vi "main.vi"() -> ()   [LabVIEW 2019]
uses:
  <vilib>/Utility/sysdir.llb/System Directory Type.ctl
  <vilib>/Platform/browser.llb/Open URL in Default Browser (string).vi
  <vilib>/Utility/cursorutil.llb/Set Cursor (Icon Pict).vi
  <vilib>/regexp/Match Regular Expression.xnode
  lib/libSimulationControl/libSimulationControl.lvlib
panel:
  out "Impressum":string
  out "Running?":bool
  in  "Help Button":bool
  in  "Break":bool
  in  "Plot":bool
  in  "Stop Button":bool
  in  "Pause Button":bool
  in  "Run":bool
  in  "Tab Control":T1(tab)
  out "Active element":string
  out "Iteration":i32
  out "Plant structure":string
  out "Simulation log":string
  in  "Auto Scroll":bool
  in  "Reset":bool
  in  "Uncouple":bool
  out "Working directory":path
  out "Runtime":dbl
  in  "Console":bool
  out "Runtime":string
  in  "Env. Clear":bool
  out "Env. Structure":string
  in  "Load Env":bool
  out "Environtment ready?":bool
  in  "Create Env":bool
  in  "Environtment Dir":path
  in  "Environment Tree":string(tree)
  out "Reactor Legend":picture
  in  "Show legend":bool
  out "Feedback?":bool
  out "Methane?":bool
  out "Storage?":bool
  out "#Hydrolysis":dbl
  out "Plant":picture
  in  "Reactor State":string(combo)="STRUCT_1_STAGE.vi"
  in  "Flow [L/h]":dbl=10.0 min=5.0 max=100.0 step=1.0
  in  "Hydrolysis specification":path
  in  "Methane specification":path
  in  "Auto cleanup?":bool
  in  "Endtime":dbl
  in  "Starttime":dbl
  in  "Edit Methane":bool
  in  "Edit Hydro":bool
  in  "Simulation file":path
  out "#Reactors":i32
  in  "Inflow fractions":T2(array[cluster]) {"Vertical Pointer Slide" scale=0.0..100.0 scale format="%.0f%"}
  in  "Hydrolysis PH":cluster{"Meter":dbl, "String":string}[][](array[cluster]) {"Meter" scale=0.0..14.0}
  in  "Load Feeding":bool
  in  "Save Feeding":bool
  out "Valid stamp?":bool
  out "Next timestep":dbl
  in  "Reactor":string(combo)
  in  "Delete":bool
  in  "Add timestamp":string[](array[string])
  in  "Add":bool
  in  "Feeding table":i32(listbox)
  out "timetable":string
  # "Biogas simulation Control"
  # "Before you start the simulation you need to set up a working environment.\nThe environment will be for the chosen reactor structure only."
  # "If you want the hydrolysis reactors to start with different initial values, you need to set up a working environtment first."
  # "Change the proportions at which the methane outflow will \nbe fed back into the hydrolysis reactors:"
  # "Add feeding hours and amount for a hydrolysis reactor."
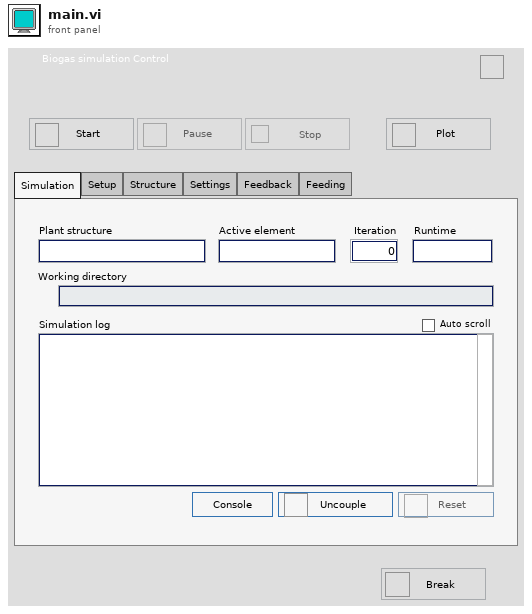
[diagram p1: front panel]
types:
  T1 = enum32{"Simulation", "Setup", "Structure", "Settings", "Feedback", "Feeding"}
  T2 = cluster{"Vertical Pointer Slide":i32, "String":string}[]
  T3 = typedef "System Directory Type.ctl" = i32
  T4 = enum8{"Enabled", "Disabled", "Disabled and Grayed Out"}
  T5 = typedef "LVPoint32TypeDef.ctl" = cluster{"Horizontal":i32, "Vertical":i32}
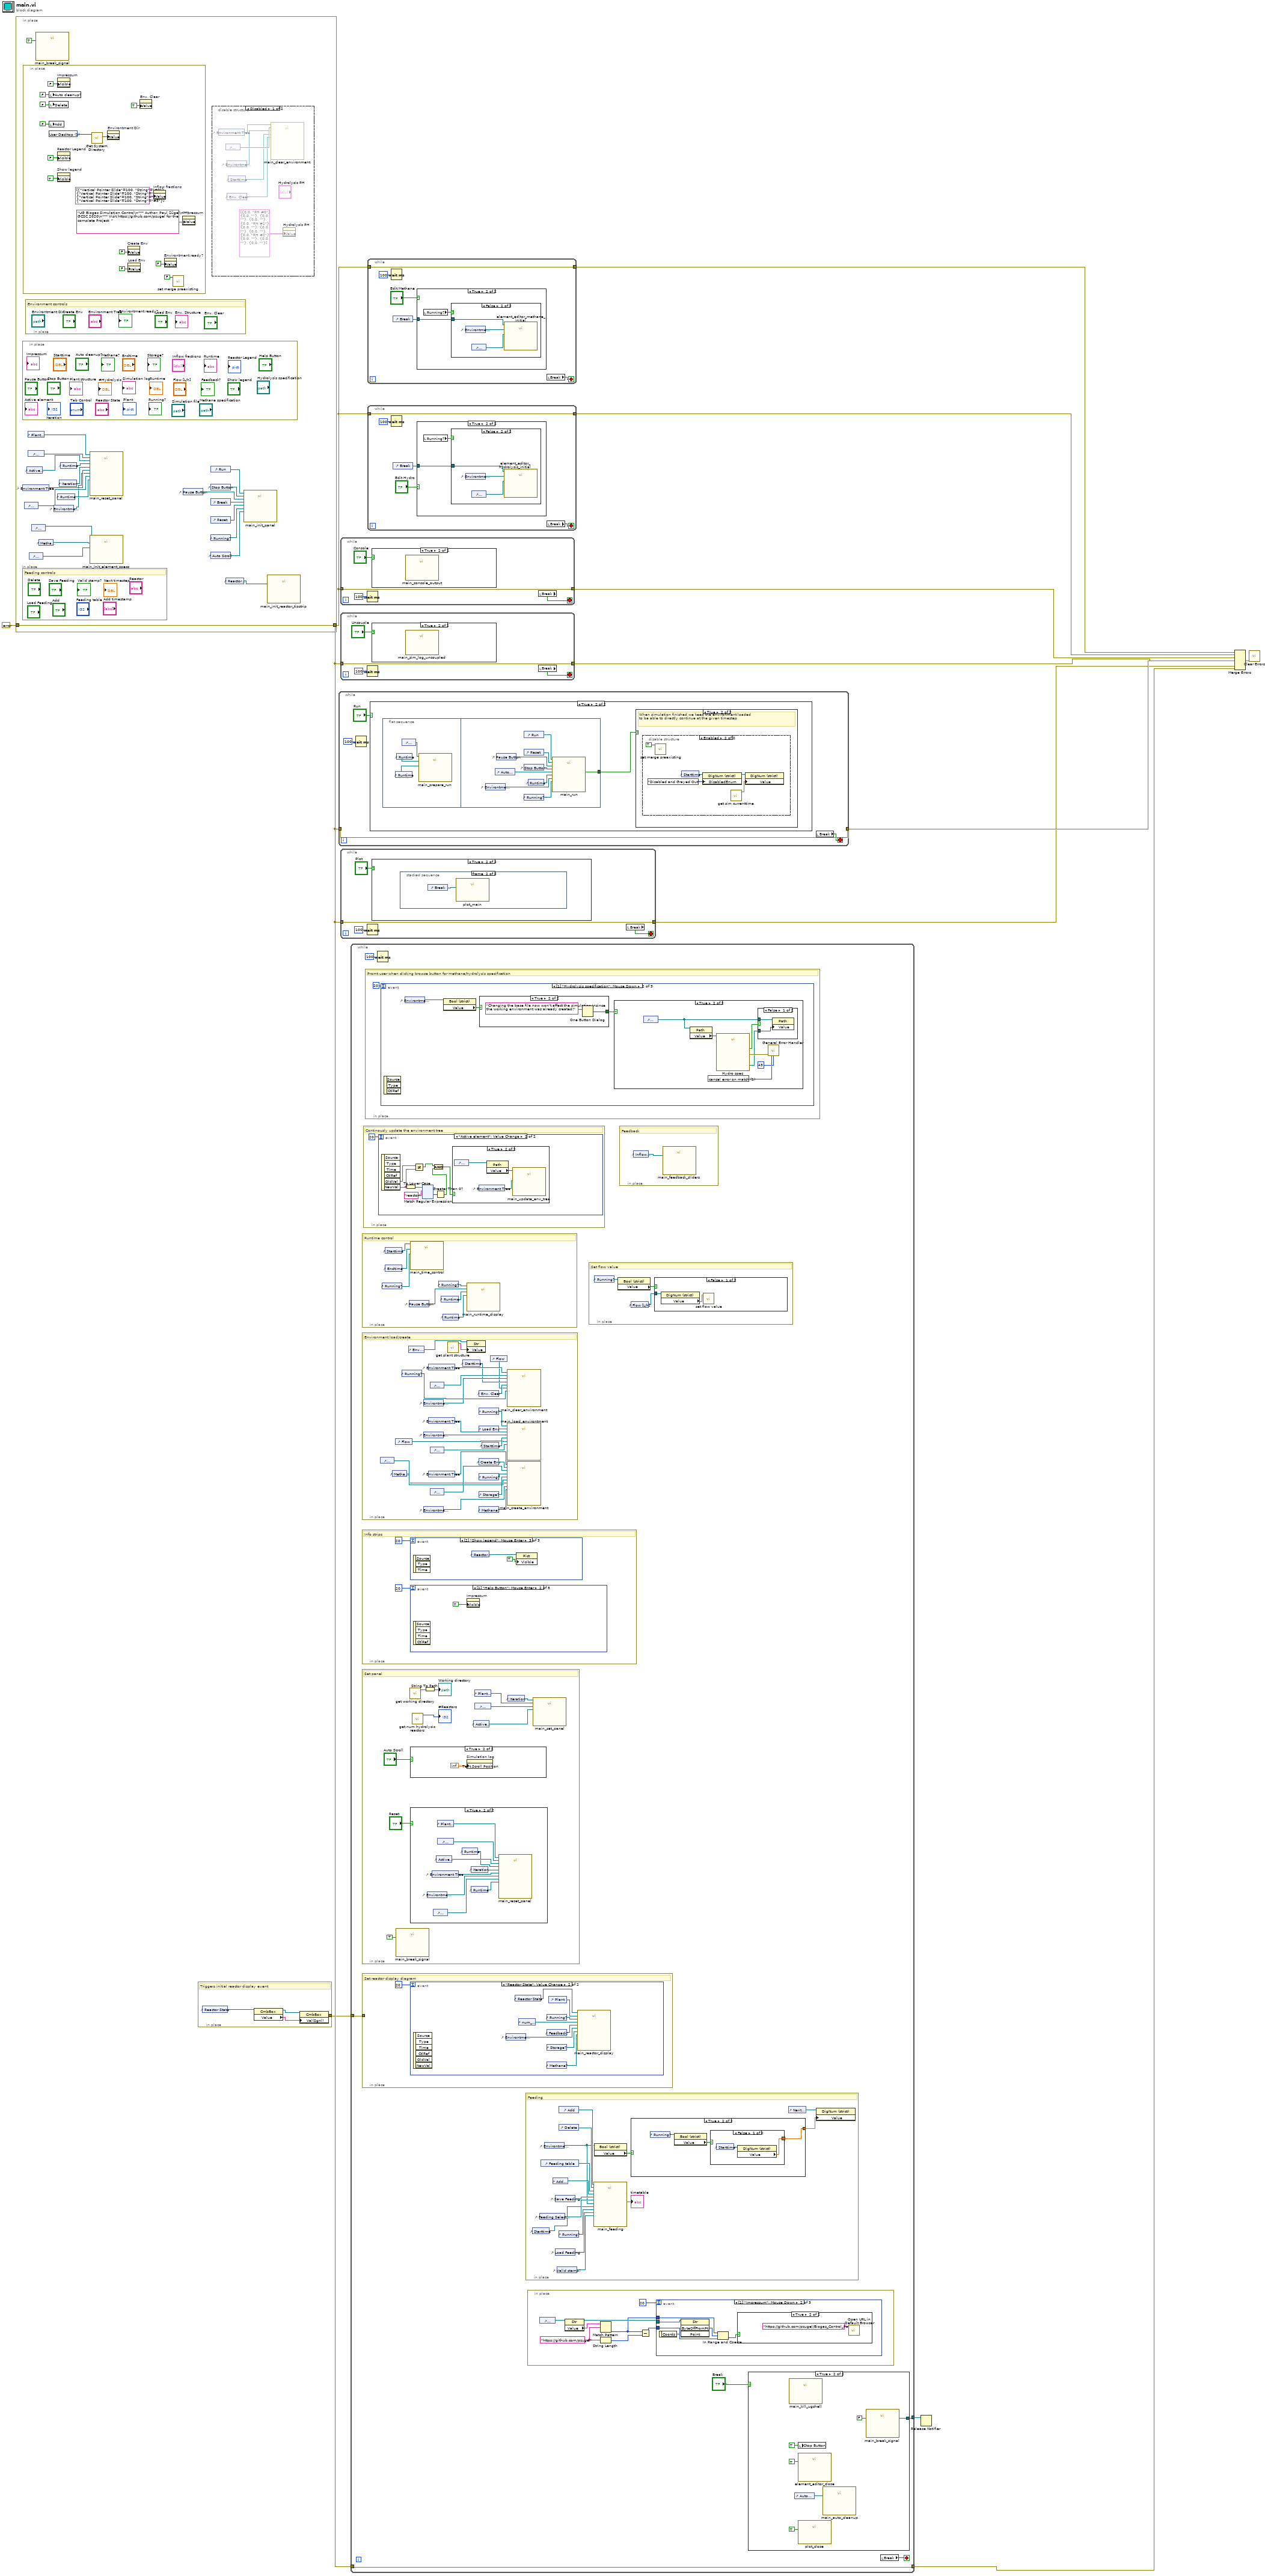
[diagram p0: block diagram]
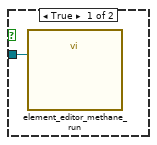
[diagram p3: hidden frame]
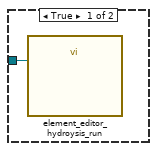
[diagram p5: hidden frame]
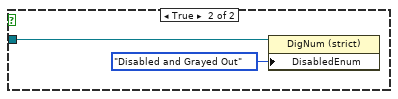
[diagram p8: hidden frame]
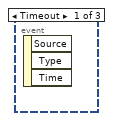
[diagram p9: hidden frame]
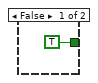
[diagram p10: hidden frame]
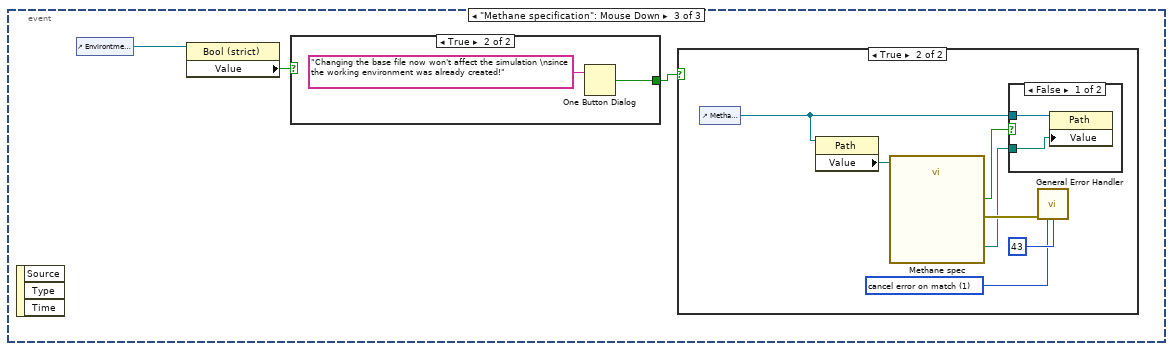
[diagram p13: hidden frame]
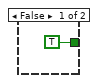
[diagram p16: hidden frame]
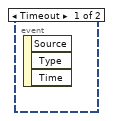
[diagram p17: hidden frame]
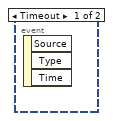
[diagram p19: hidden frame]
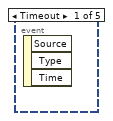
[diagram p20: hidden frame]
diagram:
  n1 = in-place {
    in-place-border: [w34] -> w5
    in-place-border: errorcluster {"status"=FALSE, "code"=0, "source"=""} ("error constant") -> [w34]
    n2 = in-place {
    }
    n3 = control-ref of="Environment Tree"() -> (w17:refnum<vi>)
    n4 = in-place {
      # "Feeding controls"
    }
    n5 = in-place {
      w46 = T3 1 items=["User Home"=0, "User Desktop"=1, "User Documents"=2, "User Application Data"=3, "User Preferences"=4, "User Temporary"=5, "Public Documents"=6, "Public Application Data"=7, "Public Preferences"=8, "Public Cache"=13, "System Core Libraries"=9, "System Installed Libraries"=10, "Application Files"=11, "Boot Volume Root"=12] ("system directory type")
      n6 = local write "Auto cleanup?"(FALSE ("Auto Cleanup?")) -> ()
      n7 = local write "Delete"(FALSE ("Delete")) -> ()
      n8 = local write "Add"(FALSE ("Add")) -> ()
      n9 = property on="Impressum" class="Str"("Visible"=FALSE) -> ()  [unwired: 2 in, 2 out]
      n10 = property on="Reactor Legend" class="Pict"("Visible"=FALSE) -> ()  [unwired: 2 in, 2 out]
      n11 = property on="Show legend" class="Bool"("Visible"=TRUE) -> ()  [unwired: 2 in, 2 out]
      n12 = call <vilib>:"Get System Directory.vi"("system directory type"=w46) -> ("system directory"=w47:path)  [unwired: 10 in]
      n13 = property on="Environtment Dir" class="Path"("Value"=w47) -> ()  [unwired: 2 in, 2 out]
      n14 = property on="Create Env" class="Bool (strict)"("Value"=FALSE ("Create Env")) -> ()  [unwired: 2 in, 2 out]
      n15 = property on="Load Env" class="Bool (strict)"("Value"=FALSE ("Load Env")) -> ()  [unwired: 2 in, 2 out]
      n16 = property on="Env. Clear" class="Bool (strict)"("Value"=TRUE ("Env. Clear")) -> ()  [unwired: 2 in, 2 out]
      n17 = property on="Inflow fractions" class="Arr (strict)"("Value"=T2 [{"Vertical Pointer Slide"=100, "String"="#0"}, {"Vertical Pointer Slide"=100, "String"="#1"}, {"Vertical Pointer Slide"=100, "String"="#2"}, {"Vertical Pointer Slide"=100, "String"="#3"}] ("Inflow fractions")) -> ()  [unwired: 2 in, 2 out]
      n18 = property on="Environtment ready?" class="Bool (strict)"("Value"=FALSE ("Environtment ready?")) -> ()  [unwired: 2 in, 2 out]
      n19 = call "set merge preexisting.vi"("merge"=FALSE) -> ()  [unwired: 10 in, 1 out]
      n20 = property on="Impressum" class="Str"("Value"="UG Biogas Simulation Control\n*** Author: Paul Zügel\n*** GCSC 2020\n*** Visit https://github.com/pzugel for the complete Project  " ("String")) -> ()  [unwired: 2 in, 2 out]
    }
    n21 = control-ref of="Environtment Dir"() -> (w18:refnum<vi>)
    n22 = in-place {
      # "Environment controls"
    }
    n23 = control-ref of="Active element"() -> (w32:refnum<vi>)
    n24 = control-ref of="Plant structure"() -> (w30:refnum<vi>)
    n25 = control-ref of="Simulation log"() -> (w31:refnum<vi>)
    n26 = control-ref of="Simulation file"() -> (w20:refnum<vi>)
    n27 = control-ref of="Hydrolysis specification"() -> (w14:refnum<vi>)
    n28 = call "main_break_signal.vi"("Keep Running?"=TRUE ("Checkbox")) -> ()  [unwired: 10 in, 1 out]
    n29 = control-ref of="Methane specification"() -> (w13:refnum<vi>)
    n30 = control-ref of="Environtment ready?"() -> (w16:refnum<vi>)
    n31 = control-ref of="Runtime"() -> (w21:refnum<vi>)
    n32 = control-ref of="Iteration"() -> (w33:refnum<vi>)
    n33 = control-ref of="Runtime"() -> (w19:refnum<vi>)
    n34 = call "main_reset_panel.vi"("Env ready?"=w16, "Envi. Tree"=w17, "Env. Directory"=w18, "Iteration"=w33, "Runtime"=w21, "Runtime (string)"=w19, "Active Element"=w32, "Simulation Log"=w31, "Plant Structure"=w30) -> ()  [unwired: 3 in]
    n35 = call "main_init_element_specs.vi"("Simulation"=w20, "Methane"=w13, "Hydrolyse"=w14) -> ()  [unwired: 9 in]
    n36 = control-ref of="Pause Button"() -> (w23:refnum<vi>)
    n37 = control-ref of="Run"() -> (w29:refnum<vi>)
    n38 = control-ref of="Stop Button"() -> (w24:refnum<vi>)
    n39 = control-ref of="Break"() -> (w27:refnum<vi>)
    n40 = control-ref of="Reset"() -> (w28:refnum<vi>)
    n41 = control-ref of="Running?"() -> (w22:refnum<vi>)
    n42 = control-ref of="Auto Scroll"() -> (w26:refnum<vi>)
    n43 = disable-structure shown="Disabled" {
      frame Disabled {
        n44 = control-ref of="Environment Tree"() -> (w40:refnum<vi>)
        n45 = control-ref of="Environtment Dir"() -> (w39:refnum<vi>)
        n46 = control-ref of="Environtment ready?"() -> (w38:refnum<vi>)
        n47 = control-ref of="Env. Clear"() -> (w36:refnum<vi>)
        n48 = control-ref of="Starttime"() -> (w37:refnum<vi>)
        n49 = call "main_clear_environment.vi"("Env. Clear"=w36, "Starttime"=w37, "Env. ready?"=w38, "Env. Dir"=w39, "Env. Tree"=w40) -> ()  [unwired: 7 in]
        n50 = property on="Hydrolysis PH" class="Arr (strict)"("Value"=cluster{"Meter":dbl, "String":string}[][] [[{"Meter"=0.0, "String"="PH #0"}, {"Meter"=0.0, "String"=""}, {"Meter"=0.0, "String"=""}, {"Meter"=0.0, "String"=""}], [{"Meter"=0.0, "String"="PH #1"}, {"Meter"=0.0, "String"=""}, {"Meter"=0.0, "String"=""}, {"Meter"=0.0, "String"=""}], [{"Meter"=0.0, "String"="PH #2"}, {"Meter"=0.0, "String"=""}, {"Meter"=0.0, "String"=""}, {"Meter"=0.0, "String"=""}]] ("Hydrolysis PH")) -> ()  [unwired: 2 in, 2 out]
      }
      frame Enabled {
      }
    }
    n51 = control-ref of="Reactor Legend"() -> (w15:refnum<vi>)
    n52 = call "main_init_panel.vi"("Running?"=w22, "Reset"=w28, "Auto Scroll"=w26, "Break Button"=w27, "Pause Button"=w23, "Stop Button"=w24, "Run"=w29) -> ()  [unwired: 5 in]
    n53 = call "main_init_reactor_tipstrip.vi"("Reactor legend"=w15) -> ()  [unwired: 11 in]
  }
  n54 = in-place {
    in-place-border: [w56] -> w1
    # "Triggers initial reactor display event"
    n55 = control-ref of="Reactor State"() -> (w59:refnum<vi>)
    n56 = property class="CmbBox"(reference=w59) -> (reference out=w57:refnum<vi>, "Value"=w58:string)  [unwired: 1 in, 1 out]
    n57 = property class="CmbBox"(reference=w57, "Val(Sgnl)"=w58) -> (error out=w56:errorcluster)  [unwired: 1 in, 1 out]
  }
  n58 = while {
    tunnel: w5 -> [w63]
    tunnel: [w63] -> w11
    stop <- w61 stop-if-true
    n59 = Wait (ms)(milliseconds to wait=u32 100) -> ()  [unwired: 1 out]
    n60 = case shown="True" "Run" {
      frame False {
        n61 = property on="Run" class="Bool"("DisabledEnum"=T4."Enabled" ("Disabled")) -> ()  [unwired: 2 in, 2 out]
        n62 = property on="Stop Button" class="Bool (strict)"("DisabledEnum"=T4."Disabled and Grayed Out" ("Disabled")) -> ()  [unwired: 2 in, 2 out]
        n63 = property on="Pause Button" class="Bool (strict)"("DisabledEnum"=T4."Disabled and Grayed Out" ("Disabled")) -> ()  [unwired: 2 in, 2 out]
      }
      frame True {
        n64 = flat-sequence {
          tunnel: [w82] -> w67
          frame #0 {
            n65 = control-ref of="Runtime"() -> (w81:refnum<vi>)
            n66 = control-ref of="Runtime"() -> (w80:refnum<vi>)
            n67 = control-ref of="Environtment Dir"() -> (w79:refnum<vi>)
            n68 = call "main_prepare_run.vi"("Runtime"=w81, "Runtime String"=w80, "Env. Dir"=w79) -> ()  [unwired: 9 in]
          }
          frame #1 {
            n69 = control-ref of="Environtment ready?"() -> (w90:refnum<vi>)
            n70 = control-ref of="Auto cleanup?"() -> (w89:refnum<vi>)
            n71 = control-ref of="Pause Button"() -> (w86:refnum<vi>)
            n72 = control-ref of="Run"() -> (w84:refnum<vi>)
            n73 = control-ref of="Reset"() -> (w88:refnum<vi>)
            n74 = control-ref of="Stop Button"() -> (w85:refnum<vi>)
            n75 = control-ref of="Running?"() -> (w87:refnum<vi>)
            n76 = control-ref of="Runtime"() -> (w83:refnum<vi>)
            n77 = call "main_run.vi"("Runtime String"=w83, "Env ready?"=w90, "Cleanup?"=w89, "Running?"=w87, "Stop Button"=w85, "Pause Button"=w86, "Reset"=w88, "Run"=w84) -> ("OK?"=w82:bool)  [unwired: 3 in]
          }
        }
        n78 = case shown="True" w67 {
          frame False {
          }
          frame True {
            # "When simulation finished we keep the environment loaded\nto be able to directly continue at the given timestep"
            n79 = disable-structure shown="Enabled" {
              frame Disabled {
                n80 = control-ref of="Env. Clear"() -> (w72:refnum<vi>)
                n81 = property class="Bool (strict)"(reference=w72, "Value"=TRUE) -> (reference out=w73:refnum<vi>)  [unwired: 1 in, 1 out]
                n82 = control-ref of="Environtment ready?"() -> (w71:refnum<vi>)
                n83 = control-ref of="Environment Tree"() -> (w69:refnum<vi>)
                n84 = control-ref of="Environtment Dir"() -> (w70:refnum<vi>)
                n85 = call "main_clear_environment.vi"("Env. Clear"=w73, "Env. ready?"=w71, "Env. Dir"=w70, "Env. Tree"=w69) -> ()  [unwired: 8 in]
              }
              frame Enabled {
                n86 = call "set merge preexisting.vi"("merge"=TRUE) -> ()  [unwired: 10 in, 1 out]
                n87 = control-ref of="Starttime"() -> (w77:refnum<vi>)
                n88 = property class="DigNum (strict)"(reference=w77, "DisabledEnum"=T4."Disabled and Grayed Out" ("Disabled")) -> (reference out=w74:refnum<vi>)  [unwired: 1 in, 1 out]
                n89 = call "get sim currenttime.vi"() -> ("current_time"=w75:dbl)  [unwired: 10 in, 1 out]
                n90 = property class="DigNum (strict)"(reference=w74, "Value"=w75) -> ()  [unwired: 1 in, 2 out]
              }
            }
          }
        }
      }
    }
    n91 = local read "Break"() -> (w61:bool)
  }
  n92 = while {
    tunnel: w5 -> [w93]
    tunnel: [w93] -> w6
    stop <- w91 stop-if-true
    n93 = Wait (ms)(milliseconds to wait=u32 100) -> ()  [unwired: 1 out]
    n94 = case shown="True" "Console" {
      frame False {
      }
      frame True {
        n95 = call "main_console_output.vi"() -> ()  [unwired: 12 in]
      }
    }
    n96 = local read "Break"() -> (w91:bool)
  }
  n97 = while {
    tunnel: w5 -> [w97]
    tunnel: [w97] -> w7
    stop <- w95 stop-if-true
    n98 = Wait (ms)(milliseconds to wait=u32 100) -> ()  [unwired: 1 out]
    n99 = case shown="True" "Uncouple" {
      frame False {
      }
      frame True {
        n100 = call "main_sim_log_uncoupled.vi"() -> ()  [unwired: 12 in]
      }
    }
    n101 = local read "Break"() -> (w95:bool)
  }
  n102 = while {
    tunnel: w5 -> [w101]
    tunnel: [w101] -> w10
    stop <- w99 stop-if-true
    n103 = Wait (ms)(milliseconds to wait=u32 100) -> ()  [unwired: 1 out]
    n104 = case shown="True" "Plot" {
      frame False {
      }
      frame True {
        n105 = stacked-sequence {
          frame #0 {
            n106 = call "plot_close.vi"("Close?"=TRUE) -> ()  [unwired: 11 in]
          }
          frame #1 {
            n107 = control-ref of="Break"() -> (w104:refnum<vi>)
            n108 = call "plot_main.vi"("Break"=w104) -> ()  [unwired: 11 in]
          }
        }
      }
    }
    n109 = local read "Break"() -> (w99:bool)
  }
  n110 = while {
    tunnel: w5 -> [w110]
    tunnel: [w110] -> w9
    tunnel: [w108] -> w8
    tunnel: w1 -> [w105]
    stop <- w106 stop-if-true
    n111 = in-place {
      # "Runtime control"
      n112 = control-ref of="Running?"() -> (w280:refnum<vi>)
      n113 = control-ref of="Starttime"() -> (w282:refnum<vi>)
      n114 = control-ref of="Endtime"() -> (w281:refnum<vi>)
      n115 = control-ref of="Pause Button"() -> (w277:refnum<vi>)
      n116 = call "main_time_control.vi"("Running?"=w280, "Endtime"=w281, "Starttime"=w282) -> ()  [unwired: 9 in]
      n117 = control-ref of="Running?"() -> (w276:refnum<vi>)
      n118 = control-ref of="Runtime"() -> (w278:refnum<vi>)
      n119 = control-ref of="Runtime"() -> (w279:refnum<vi>)
      n120 = call "main_runtime_display.vi"("Runtime (string)"=w279, "Runtime"=w278, "Pause Button"=w277, "Running?"=w276) -> ()  [unwired: 8 in]
    }
    n121 = in-place {
      # "Environment load/create"
      n122 = control-ref of="Hydrolysis specification"() -> (w327:refnum<vi>)
      n123 = control-ref of="Methane specification"() -> (w326:refnum<vi>)
      n124 = control-ref of="Flow"() -> (w324:refnum<vi>)
      n125 = control-ref of="Running?"() -> (w325:refnum<vi>)
      n126 = control-ref of="Env. Structure"() -> (w337:refnum<vi>)
      n127 = control-ref of="Environtment ready?"() -> (w333:refnum<vi>)
      n128 = control-ref of="Environtment ready?"() -> (w336:refnum<vi>)
      n129 = control-ref of="Environtment ready?"() -> (w341:refnum<vi>)
      n130 = control-ref of="Environment Tree"() -> (w331:refnum<vi>)
      n131 = control-ref of="Environment Tree"() -> (w338:refnum<vi>)
      n132 = control-ref of="Environment Tree"() -> (w347:refnum<vi>)
      n133 = control-ref of="Environtment Dir"() -> (w332:refnum<vi>)
      n134 = control-ref of="Environtment Dir"() -> (w335:refnum<vi>)
      n135 = control-ref of="Environtment Dir"() -> (w345:refnum<vi>)
      n136 = call "get plant structure.vi"() -> ("function return"=w329:string)  [unwired: 10 in, 1 out]
      n137 = control-ref of="Starttime"() -> (w328:refnum<vi>)
      n138 = property class="Str"(reference=w337, "Value"=w329) -> ()  [unwired: 1 in, 2 out]
      n139 = control-ref of="Env. Clear"() -> (w334:refnum<vi>)
      n140 = control-ref of="Running?"() -> (w340:refnum<vi>)
      n141 = control-ref of="Load Env"() -> (w339:refnum<vi>)
      n142 = control-ref of="Create Env"() -> (w346:refnum<vi>)
      n143 = control-ref of="Running?"() -> (w344:refnum<vi>)
      n144 = control-ref of="Storage?"() -> (w343:refnum<vi>)
      n145 = control-ref of="Methane?"() -> (w342:refnum<vi>)
      n146 = control-ref of="Starttime"() -> (w330:refnum<vi>)
      n147 = control-ref of="Flow"() -> (w323:refnum<vi>)
      n148 = call "main_clear_environment.vi"("Flow"=w323, "Env. Clear"=w334, "Running?"=w325, "Starttime"=w328, "Env. ready?"=w333, "Env. Dir"=w332, "Env. Tree"=w331) -> ()  [unwired: 5 in]
      n149 = call "main_load_environtment.vi"("Flow"=w324, "Starttime"=w330, "Env. Dir"=w335, "Env. Ready?"=w336, "Environtment Tree"=w338, "Load Env"=w339, "Running?"=w340) -> ()  [unwired: 5 in]
      n150 = call "main_create_environment.vi"("Meth. Path"=w326, "Hydr. Path"=w327, "Ready?"=w341, "Storage?"=w343, "Methane?"=w342, "Running?"=w344, "Directory"=w345, "Create"=w346, "Environtment Tree"=w347) -> ()  [unwired: 3 in]
    }
    n151 = in-place {
      # "Info strips"
      n152 = event shown="[2] \"Show legend\": Mouse Enter" {
        selector: _ -> [_ _ _]
        dyn-events: _ -> [_ _ _]
        timeout: 20 -> [_ _ _]
        event Timeout {
          n153 = event-data() -> ()  [unwired: 1 in, 3 out]
        }
        event "Show legend": Mouse Leave {
          n154 = event-data() -> ()  [unwired: 1 in, 3 out]
          n155 = control-ref of="Reactor Legend"() -> (w300:refnum<vi>)
          n156 = property class="Pict"(reference=w300, "Visible"=FALSE) -> ()  [unwired: 1 in, 2 out]
        }
        event "Show legend": Mouse Enter {
          n157 = event-data() -> ()  [unwired: 1 in, 3 out]
          n158 = control-ref of="Reactor Legend"() -> (w302:refnum<vi>)
          n159 = property class="Pict"(reference=w302, "Visible"=TRUE) -> ()  [unwired: 1 in, 2 out]
        }
      }
      n160 = event shown="[1] \"Help Button\": Mouse Enter" {
        selector: _ -> [_ _ _ _ _]
        dyn-events: _ -> [_ _ _ _ _]
        timeout: 20 -> [_ _ _ _ _]
        event Timeout {
          n161 = event-data() -> ()  [unwired: 1 in, 3 out]
        }
        event "Help Button": Mouse Enter {
          n162 = event-data() -> ()  [unwired: 1 in, 4 out]
          n163 = property on="Impressum" class="Str"("Visible"=TRUE) -> ()  [unwired: 2 in, 2 out]
        }
        event "Help Button": Mouse Leave {
          n164 = event-data() -> ()  [unwired: 1 in, 4 out]
          n165 = event shown="[0] Timeout" {
            selector: _ -> [_ _]
            dyn-events: _ -> [_ _]
            timeout: 20 -> [_ _]
            event Timeout {
              n166 = event-data() -> ()  [unwired: 1 in, 3 out]
              n167 = property on="Impressum" class="Str"("Visible"=FALSE) -> ()  [unwired: 2 in, 2 out]
            }
            event "Impressum": Mouse Enter {
              n168 = event-data() -> ()  [unwired: 1 in, 3 out]
              n169 = property on="Impressum" class="Str"("Visible"=TRUE) -> ()  [unwired: 2 in, 2 out]
            }
          }
        }
        event "Impressum": Mouse Enter {
          n170 = event-data() -> ()  [unwired: 1 in, 4 out]
        }
        event "Impressum": Mouse Leave {
          n171 = event-data() -> ()  [unwired: 1 in, 4 out]
          n172 = property on="Impressum" class="Str"("Visible"=FALSE) -> ()  [unwired: 2 in, 2 out]
        }
      }
    }
    n173 = in-place {
      # "Set panel"
      n174 = call "main_break_signal.vi"("Keep Running?"=TRUE) -> ()  [unwired: 10 in, 1 out]
      n175 = call "get working directory.vi"() -> ("function return"=w312:string)  [unwired: 10 in, 1 out]
      n176 = case shown="True" "Auto Scroll" {
        frame False {
        }
        frame True {
          n177 = property on="Simulation log" class="Str"("Text.Scroll Position"=inf) -> ()  [unwired: 2 in, 2 out]
        }
      }
      n178 = case shown="True" "Reset" {
        frame False {
        }
        frame True {
          n179 = control-ref of="Environtment ready?"() -> (w314:refnum<vi>)
          n180 = control-ref of="Environment Tree"() -> (w315:refnum<vi>)
          n181 = control-ref of="Environtment Dir"() -> (w316:refnum<vi>)
          n182 = control-ref of="Active element"() -> (w320:refnum<vi>)
          n183 = control-ref of="Plant structure"() -> (w321:refnum<vi>)
          n184 = control-ref of="Simulation log"() -> (w318:refnum<vi>)
          n185 = control-ref of="Runtime"() -> (w313:refnum<vi>)
          n186 = control-ref of="Iteration"() -> (w319:refnum<vi>)
          n187 = control-ref of="Runtime"() -> (w317:refnum<vi>)
          n188 = call "main_reset_panel.vi"("Env ready?"=w314, "Envi. Tree"=w315, "Env. Directory"=w316, "Iteration"=w319, "Runtime"=w317, "Runtime (string)"=w313, "Active Element"=w320, "Simulation Log"=w318, "Plant Structure"=w321) -> ()  [unwired: 3 in]
        }
      }
      n189 = call "get num hydrolysis reactors.vi"() -> ("function return"=→"#Reactors":i32)  [unwired: 10 in, 1 out]
      n190 = String To Path(string=w312) -> (path=→"Working directory":path)
      n191 = control-ref of="Active element"() -> (w306:refnum<vi>)
      n192 = control-ref of="Plant structure"() -> (w304:refnum<vi>)
      n193 = control-ref of="Simulation log"() -> (w305:refnum<vi>)
      n194 = control-ref of="Iteration"() -> (w303:refnum<vi>)
      n195 = call "main_set_panel.vi"("Active Element"=w306, "Simulation Log"=w305, "Plant Structure"=w304, "Iteration"=w303) -> ()  [unwired: 8 in]
    }
    n196 = in-place {
      in-place-border: w105 -> [_]
      # "Set reactor display diagram"
      n197 = event shown="[1] \"Reactor State\": Value Change" {
        selector: _ -> [_ _]
        dyn-events: _ -> [_ _]
        timeout: 20 -> [_ _]
        event Timeout {
          n198 = event-data() -> ()  [unwired: 1 in, 3 out]
        }
        event "Reactor State": Value Change {
          n199 = event-data() -> ()  [unwired: 1 in, 6 out]
          n200 = control-ref of="Environtment ready?"() -> (w291:refnum<vi>)
          n201 = control-ref of="Reactor State"() -> (w284:refnum<vi>)
          n202 = control-ref of="num_Hydrolysis"() -> (w287:refnum<vi>)
          n203 = control-ref of="Running?"() -> (w286:refnum<vi>)
          n204 = control-ref of="Feedback?"() -> (w290:refnum<vi>)
          n205 = control-ref of="Storage?"() -> (w288:refnum<vi>)
          n206 = control-ref of="Methane?"() -> (w289:refnum<vi>)
          n207 = control-ref of="Plant"() -> (w285:refnum<vi>)
          n208 = call "main_reactor_display.vi"("Env. Ready?"=w291, "Storage?"=w288, "Feedback?"=w290, "Methane?"=w289, "#Hydrolysis"=w287, "Running?"=w286, "Plant Picture"=w285, "Reactor State"=w284) -> ()  [unwired: 4 in]
        }
      }
    }
    n209 = in-place {
      # "Continously update the environment tree"
      n210 = event shown="[1] \"Active element\": Value Change" {
        selector: _ -> [_ _]
        dyn-events: _ -> [_ _]
        timeout: 20 -> [_ _]
        event Timeout {
          n211 = event-data() -> ()  [unwired: 1 in, 3 out]
        }
        event "Active element": Value Change {
          n212 = event-data() -> ("OldVal"=w154:string, "NewVal"=w153:string)  [unwired: 1 in, 4 out]
          n213 = To Lower Case(string=w153) -> (all lower case string=w156:string)
          n214 = Not Equal?(x=w154, y=w153) -> (x != y?=w152:bool)
          n215 = xnode "Match Regular Expression"("input string"=w156, "regular expression"="reactor") -> ("offset past match"=w157:i32)  [unwired: 4 in, 4 out]
          n216 = Greater Than 0?(x=w157) -> (x > 0?=w151:bool)
          n217 = And(x=w152, y=w151) -> (x .and. y?=w150:bool)
          n218 = case shown="True" w150 {
            frame False {
            }
            frame True {
              n219 = control-ref of="Environtment Dir"() -> (w159:refnum<vi>)
              n220 = control-ref of="Environment Tree"() -> (w160:refnum<vi>)
              n221 = property class="Path"(reference=w159) -> ("Value"=w158:path)  [unwired: 1 in, 2 out]
              n222 = call "main_update_env_tree.vi"("Env. Tree"=w160, "Env_path"=w158) -> ()  [unwired: 10 in]
            }
          }
        }
      }
    }
    n223 = in-place {
      # "Promt user when clicking browse button for methane/hydrolysis specification"
      n224 = event shown="[1] \"Hydrolysis specification\": Mouse Down" {
        selector: _ -> [_ _ _]
        dyn-events: _ -> [_ _ _]
        timeout: 20 -> [_ _ _]
        event Timeout {
          n225 = event-data() -> ()  [unwired: 1 in, 3 out]
        }
        event "Hydrolysis specification": Mouse Down {
          n226 = event-data() -> ()  [unwired: 1 in, 3 out]
          n227 = control-ref of="Environtment ready?"() -> (w121:refnum<vi>)
          n228 = property class="Bool (strict)"(reference=w121) -> ("Value"=w120:bool)  [unwired: 1 in, 2 out]
          n229 = case shown="True" w120 {
            tunnel: [TRUE ("true") w123] -> w119
            frame False {
            }
            frame True {
              n230 = One Button Dialog(message="Changing the base file now won't affect the simulation \nsince the working environment was already created!") -> (true=w123:bool)  [unwired: 1 in]
            }
          }
          n231 = case shown="True" w119 {
            frame False {
            }
            frame True {
              w129 = 1 items=["no exception", "cancel error on match", "set error on match"] ("[exception action] (none:0)")
              n232 = control-ref of="Hydrolysis specification"() -> (w127:refnum<vi>)
              n233 = property class="Path"(reference=w127) -> ("Value"=w128:path)  [unwired: 1 in, 2 out]
              n234 = call "Hydro spec"("start path"=w128) -> ("selected path"=w126:path, "cancelled"=w125:bool, "error out"=w130:errorcluster)  [unwired: 11 in, 1 out]
              n235 = case shown="False" w125 {
                tunnel: w127 -> [w133 _]
                tunnel: w126 -> [w132 _]
                frame False {
                  n236 = property class="Path"(reference=w133, "Value"=w132) -> ()  [unwired: 1 in, 2 out]
                }
                frame True {
                }
              }
              n237 = call <vilib>:"General Error Handler.vi"("error in (no error)"=w130, "[exception action] (none:0)"=w129, "[exception code]"=43) -> ()  [unwired: 8 in, 5 out]
            }
          }
        }
        event "Methane specification": Mouse Down {
          n238 = event-data() -> ()  [unwired: 1 in, 3 out]
          n239 = control-ref of="Environtment ready?"() -> (w135:refnum<vi>)
          n240 = property class="Bool (strict)"(reference=w135) -> ("Value"=w136:bool)  [unwired: 1 in, 2 out]
          n241 = case shown="True" w136 {
            tunnel: [TRUE ("true") w147] -> w134
            frame False {
            }
            frame True {
              n242 = One Button Dialog(message="Changing the base file now won't affect the simulation \nsince the working environment was already created!") -> (true=w147:bool)  [unwired: 1 in]
            }
          }
          n243 = case shown="True" w134 {
            frame False {
            }
            frame True {
              w141 = 1 items=["no exception", "cancel error on match", "set error on match"] ("[exception action] (none:0)")
              n244 = control-ref of="Methane specification"() -> (w137:refnum<vi>)
              n245 = property class="Path"(reference=w137) -> ("Value"=w140:path)  [unwired: 1 in, 2 out]
              n246 = call "Methane spec"("start path"=w140) -> ("selected path"=w139:path, "cancelled"=w138:bool, "error out"=w142:errorcluster)  [unwired: 11 in, 1 out]
              n247 = case shown="False" w138 {
                tunnel: w137 -> [w145 _]
                tunnel: w139 -> [w144 _]
                frame False {
                  n248 = property class="Path"(reference=w145, "Value"=w144) -> ()  [unwired: 1 in, 2 out]
                }
                frame True {
                }
              }
              n249 = call <vilib>:"General Error Handler.vi"("error in (no error)"=w142, "[exception action] (none:0)"=w141, "[exception code]"=43) -> ()  [unwired: 8 in, 5 out]
            }
          }
        }
      }
    }
    n250 = Wait (ms)(milliseconds to wait=u32 100) -> ()  [unwired: 1 out]
    n251 = in-place {
      # "Feeding"
      n252 = control-ref of="Starttime"() -> (w348:refnum<vi>)
      n253 = control-ref of="Feeding Select Reactor"() -> (w354:refnum<vi>)
      n254 = control-ref of="Feeding table"() -> (w362:refnum<vi>)
      n255 = control-ref of="Environtment ready?"() -> (w349:refnum<vi>)
      n256 = control-ref of="Add timestamp"() -> (w361:refnum<vi>)
      n257 = control-ref of="Save Feeding"() -> (w356:refnum<vi>)
      n258 = control-ref of="Load Feeding"() -> (w355:refnum<vi>)
      n259 = control-ref of="Valid stamp?"() -> (w358:refnum<vi>)
      n260 = control-ref of="Add"() -> (w360:refnum<vi>)
      n261 = control-ref of="Delete"() -> (w359:refnum<vi>)
      n262 = control-ref of="Running?"() -> (w352:refnum<vi>)
      n263 = call "main_feeding.vi"("Env. Ready?"=w349, "Starttime"=w348, "Running?"=w352, "Selector"=w354, "Load"=w355, "Save"=w356, "Valid?"=w358, "New Element"=w361, "Feeding"=w362, "Delete"=w359, "Add"=w360) -> ("timetable"=→"timetable":string)
      n264 = property class="Bool (strict)"(reference=w349) -> ("Value"=w353:bool)  [unwired: 1 in, 2 out]
      n265 = case shown="True" w353 {
        tunnel: [nan w364] -> w351
        frame False {
        }
        frame True {
          n266 = control-ref of="Running?"() -> (w366:refnum<vi>)
          n267 = property class="Bool (strict)"(reference=w366) -> ("Value"=w365:bool)  [unwired: 1 in, 2 out]
          n268 = case shown="False" w365 {
            tunnel: [w367 w369] -> w364
            frame False {
              n269 = control-ref of="Starttime"() -> (w368:refnum<vi>)
              n270 = property class="DigNum (strict)"(reference=w368) -> ("Value"=w367:dbl)  [unwired: 1 in, 2 out]
            }
            frame True {
              n271 = call "get sim currenttime.vi"() -> ("current_time"=w370:dbl)  [unwired: 10 in, 1 out]
              n272 = Increment(x=w370) -> (x+1=w369:dbl)
            }
          }
        }
      }
      n273 = control-ref of="Next timestep"() -> (w350:refnum<vi>)
      n274 = property class="DigNum (strict)"(reference=w350, "Value"=w351) -> ()  [unwired: 1 in, 2 out]
    }
    n275 = in-place {
      w374 = "https://github.com/pzugel" ("regular expression")
      n276 = control-ref of="Impressum"() -> (w371:refnum<vi>)
      n277 = property class="Str"(reference=w371) -> (reference out=w378:refnum<vi>, "Value"=w373:string)  [unwired: 1 in, 1 out]
      n278 = Match Pattern(string=w373, regular expression=w374) -> (offset past match=w376:i32)  [unwired: 1 in, 3 out]
      n279 = String Length(string=w374) -> (length=w372:i32)
      n280 = Subtract(x=w376, y=w372) -> (x-y=w375:i32)
      n281 = event shown="[1] \"Impressum\": Mouse Down" {
        selector: _ -> [_ _ _]
        dyn-events: _ -> [_ _ _]
        timeout: 20 -> [_ _ _]
        tunnel: w375 -> [_ w382 w389]
        tunnel: w376 -> [_ w383 w390]
        tunnel: w378 -> [_ w380 w387]
        event Timeout {
          n282 = event-data() -> ()  [unwired: 1 in, 3 out]
        }
        event "Impressum": Mouse Down {
          n283 = event-data() -> ("Coords"=w379:T5)  [unwired: 1 in]
          n284 = invoke class="Str" method="ByteOffFromPt"(reference=w380, "Point"=w379) -> ("ByteOffFromPt"=w384:i32)  [unwired: 2 in, 3 out]
          n285 = In Range and Coerce(upper limit=w383, x=w384, lower limit=w382) -> (In Range?=w381:bool)  [unwired: 1 out]
          n286 = case shown="True" w381 {
            frame False {
            }
            frame True {
              n287 = call-poly <vilib>:"Open URL in Default Browser.vi"("URL"="https://github.com/pzugel/Biogas_Control_Panel") -> ()  [unwired: 5 in, 2 out]
            }
          }
        }
        event "Impressum": Mouse Move {
          n288 = event-data() -> ("Coords"=w386:T5)  [unwired: 1 in]
          n289 = invoke class="Str" method="ByteOffFromPt"(reference=w387, "Point"=w386) -> ("ByteOffFromPt"=w391:i32)  [unwired: 2 in, 3 out]
          n290 = In Range and Coerce(upper limit=w390, x=w391, lower limit=w389) -> (In Range?=w388:bool)  [unwired: 1 out]
          n291 = case shown="True" w388 {
            frame False {
              n292 = call-poly <vilib>:"Set Cursor.vi"("icon"=u16 1) -> ()  [unwired: 9 in, 2 out]
            }
            frame True {
              n293 = call-poly <vilib>:"Set Cursor.vi"("icon"=u16 6) -> ()  [unwired: 9 in, 2 out]
            }
          }
        }
      }
    }
    n294 = in-place "In Place Element Structure" {
      # "Set flow value"
      n295 = control-ref of="Running?"() -> (w113:refnum<vi>)
      n296 = property class="Bool (strict)"(reference=w113) -> ("Value"=w112:bool)  [unwired: 1 in, 2 out]
      n297 = control-ref of="Flow [L/h]"() -> (w111:refnum<vi>)
      n298 = case shown="False" w112 {
        tunnel: w111 -> [w114 w116]
        frame False {
          n299 = property class="DigNum (strict)"(reference=w114) -> ("Value"=w115:dbl)  [unwired: 1 in, 2 out]
          n300 = call "set flow value.vi"("val"=w115) -> ()  [unwired: 10 in, 1 out]
        }
        frame True {
          n301 = property class="DigNum (strict)"(reference=w116, "DisabledEnum"=T4."Disabled and Grayed Out" ("Disabled")) -> ()  [unwired: 1 in, 2 out]
        }
      }
    }
    n302 = in-place {
      # "Feedback"
      n303 = control-ref of="Inflow fractions"() -> (w275:refnum<vi>)
      n304 = call "main_feedback_sliders.vi"("Inflow fractions"=w275) -> ()  [unwired: 11 in]
    }
    n305 = case shown="True" "Break" {
      tunnel: [w395 w397] -> w108
      frame False {
        n306 = call "main_break_signal.vi"("Keep Running?"=TRUE ("Checkbox")) -> ("Break Notifier"=w395:refnum<notifier>)  [unwired: 10 in]
      }
      frame True {
        n307 = call "main_kill_ugshell.vi"() -> ()  [unwired: 12 in]
        n308 = control-ref of="Auto cleanup?"() -> (w396:refnum<vi>)
        n309 = local write "Stop Button"(TRUE ("Stop Button")) -> ()
        n310 = call "element_editor_close.vi"("Close?"=TRUE ("Checkbox")) -> ()  [unwired: 11 in]
        n311 = call "plot_close.vi"("Close?"=TRUE) -> ()  [unwired: 11 in]
        n312 = call "main_auto_cleanup.vi"("Cleanup?"=w396) -> ()  [unwired: 11 in]
        n313 = call "main_break_signal.vi"("Keep Running?"=FALSE ("Checkbox")) -> ("Break Notifier"=w397:refnum<notifier>)  [unwired: 10 in]
      }
    }
    n314 = local read "Break"() -> (w106:bool)
  }
  n315 = while {
    tunnel: w5 -> [w405]
    tunnel: [w405] -> w3
    stop <- w402 stop-if-true
    n316 = Wait (ms)(milliseconds to wait=u32 100) -> ()  [unwired: 1 out]
    n317 = control-ref of="Break"() -> (w403:refnum<vi>)
    n318 = case shown="True" "Edit Methane" {
      tunnel: w403 -> [_ w408]
      frame False {
      }
      frame True {
        n319 = local read "Running?"() -> (w407:bool)
        n320 = case shown="False" w407 {
          tunnel: w408 -> [w409 w412]
          frame True {
            n321 = call "element_editor_methane_run.vi"("Break"=w409) -> ()  [unwired: 11 in]
          }
          frame False {
            n322 = control-ref of="Environtment ready?"() -> (w411:refnum<vi>)
            n323 = control-ref of="Environtment Dir"() -> (w410:refnum<vi>)
            n324 = call "element_editor_methane_initial.vi"("Env. Dir"=w410, "Env. Ready?"=w411, "Break"=w412) -> ()  [unwired: 9 in]
          }
        }
      }
    }
    n325 = local read "Break"() -> (w402:bool)
  }
  n326 = while {
    tunnel: w5 -> [w417]
    tunnel: [w417] -> w4
    stop <- w413 stop-if-true
    n327 = Wait (ms)(milliseconds to wait=u32 100) -> ()  [unwired: 1 out]
    n328 = control-ref of="Break"() -> (w414:refnum<vi>)
    n329 = case shown="True" "Edit Hydro" {
      tunnel: w414 -> [_ w418]
      frame False {
      }
      frame True {
        n330 = local read "Running?"() -> (w419:bool)
        n331 = case shown="False" w419 {
          tunnel: w418 -> [w420 w421]
          frame True {
            n332 = call "element_editor_hydroysis_run.vi"("Break"=w420) -> ()  [unwired: 11 in]
          }
          frame False {
            n333 = control-ref of="Environtment ready?"() -> (w423:refnum<vi>)
            n334 = control-ref of="Environtment Dir"() -> (w422:refnum<vi>)
            n335 = call "element_editor_hydrolysis_initial.vi"("Env. Dir"=w422, "Env. Ready?"=w423, "Break"=w421) -> ()  [unwired: 9 in]
          }
        }
      }
    }
    n336 = local read "Break"() -> (w413:bool)
  }
  n337 = Release Notifier(notifier=w8) -> ()  [unwired: 2 in, 3 out]
  n338 = Merge Errors(w3, w4, w6, w7, w11, w10, w9) -> (w2:errorcluster)
  n339 = call <vilib>:"Clear Errors.vi"("error in (no error)"=w2) -> ()  [unwired: 5 in, 2 out]
